vi "GUI_HTT_MultiCamDriveDepletion.vi"() -> ()   [LabVIEW 2020]
uses:
  Shared/GUI_Template/GUI_master/tcp_new_data_event.ctl
  Shared/GUI_Template/GUI_master/tcp new data cluster.ctl
  General GUIs/Device GUIs/GUI_Cameras/Controls/Crosshair type def.ctl
  <userlib>/_OpenG.lib/array/array.llb/Filter 1D Array with Scalar (String)__ogtk.vi
panel:
  out "image1 3":T1(plugin-control)
  out "image1 2":T1(plugin-control)
  out "image1":T1(plugin-control)
  out "String 3":string="x1\ny1\nx2\ny2"
  out "String 2":string="x1\ny1\nx2\ny2"
  out "String":string="x1\ny1\nx2\ny2"
  in  "visibility":bool=TRUE
  out "appended array":string[](array[string]) caption="XH"
  out "appended array 6":string[](array[string]) caption="XH"
  out "appended array 4":string[](array[string]) caption="XH"
  in  "UDP error message":string
  out "tcp data event 2":T2
  out "error IO 2":errorcluster
  in  "Color Box":u32(colorbox)
  in  "TargetSize.Y::4":dbl=45.0 caption="y" min=2.0 max=3000.0 format="%#_6f"
  in  "TargetSize.X::4":dbl=47.0 caption="x" min=2.0 max=3000.0 format="%#_6f"
  in  "TargetSize.Y::3":dbl=163.0 caption="y" min=2.0 max=3000.0 format="%#_6f"
  in  "TargetSize.X::3":dbl=152.0 caption="x" min=2.0 max=3000.0 format="%#_6f"
  in  "TargetSize.Y::2":dbl=74.0 caption="y" min=2.0 max=3000.0 format="%#_6f"
  in  "TargetSize.X::2":dbl=75.0 caption="x" min=2.0 max=3000.0 format="%#_6f"
  in  "active cams":string
  out "CCDs":string[](array[string])
  out "Cameras":T3
  in  "Target.Y::4":dbl=45.0 caption="y" min=0.0 max=2000.0 format="%#_6f"
  in  "Target.X::4":dbl=47.0 caption="x" min=0.0 max=2000.0 format="%#_6f"
  in  "Target.Y::3":dbl=163.0 caption="y" min=0.0 max=2000.0 format="%#_6f"
  in  "Target.X::3":dbl=152.0 caption="x" min=0.0 max=2000.0 format="%#_6f"
  in  "Target.Y::2":dbl=74.0 caption="y" min=0.0 max=2000.0 format="%#_6f"
  in  "Target.X::2":dbl=75.0 caption="x" min=0.0 max=2000.0 format="%#_6f"
  out "error out":errorcluster
  in  "triggerdelay::4":dbl=0.001 caption="triggerdelay" min=0.0 max=1000000.0 format="%_4p"
  in  "triggerdelay::3":dbl=0.001 caption="triggerdelay" min=0.0 max=1000000.0 format="%_4p"
  in  "triggerdelay::2":dbl=0.001 caption="triggerdelay" min=0.0 max=100000.0 format="%_4p"
  in  "centroidy::5":dbl=0.001 caption="centroid y" min=0.0 max=0.0 format="%_4f"
  in  "centroidx::5":dbl=0.001 caption="centroid x" min=0.0 max=0.0 format="%_4f"
  in  "trigger::4":bool caption="Trigger"
  in  "centroidy::4":dbl=0.001 caption="centroid y" min=0.0 max=0.0 format="%_4f"
  in  "centroidx::4":dbl=0.001 caption="centroid x" min=0.0 max=0.0 format="%_4f"
  in  "exposure::4":dbl=0.001 caption="exposure" min=0.0 max=1000000.0 format="%_4p"
  out "image::4":T1(plugin-control) caption="HTT-MagCam-02"
  in  "GUIdevice 4":string="BellaCam24_4_dep4"
  in  "trigger::3":bool caption="Trigger"
  in  "centroidy::3":dbl=0.001 caption="centroid y" min=0.0 max=0.0 format="%_4f"
  in  "centroidx::3":dbl=0.001 caption="centroid x" min=0.0 max=0.0 format="%_4f"
  in  "exposure::3":dbl=0.001 caption="exposure" min=0.0001 max=1.0 format="%_4p"
  out "image::3":T1(plugin-control) caption="HTT-MagCam-03"
  in  "GUIdevice 3":string="BellaCam13_2_dep3"
  in  "trigger::2":bool caption="Trigger"
  in  "centroidy::2":dbl=0.001 caption="centroid y" min=0.0 max=0.0 format="%_4f"
  in  "centroidx::2":dbl=0.001 caption="centroid x" min=0.0 max=0.0 format="%_4f"
  in  "exposure::2":dbl=0.001 caption="exposure" min=1e-05 max=1.0 format="%_4p"
  out "image::2":T1(plugin-control) caption="HTT-MagCam-04"
  in  "GUIdevice 2":string="BellaCam24_2_dep2"
  out "tcp data event":T2
  in  "Refresh Button":bool caption="Update Crosshairs"
  in  "Select device":string(combo)="FrogHPD"
  in  "stop":bool
  in  "GUIdevice 1":string="HPD_CCD"
  # "XHair location"
  # "XHair location"
  # "XHair size"
  # "XHair size"
  # "XHair location"
  # "XHair size"
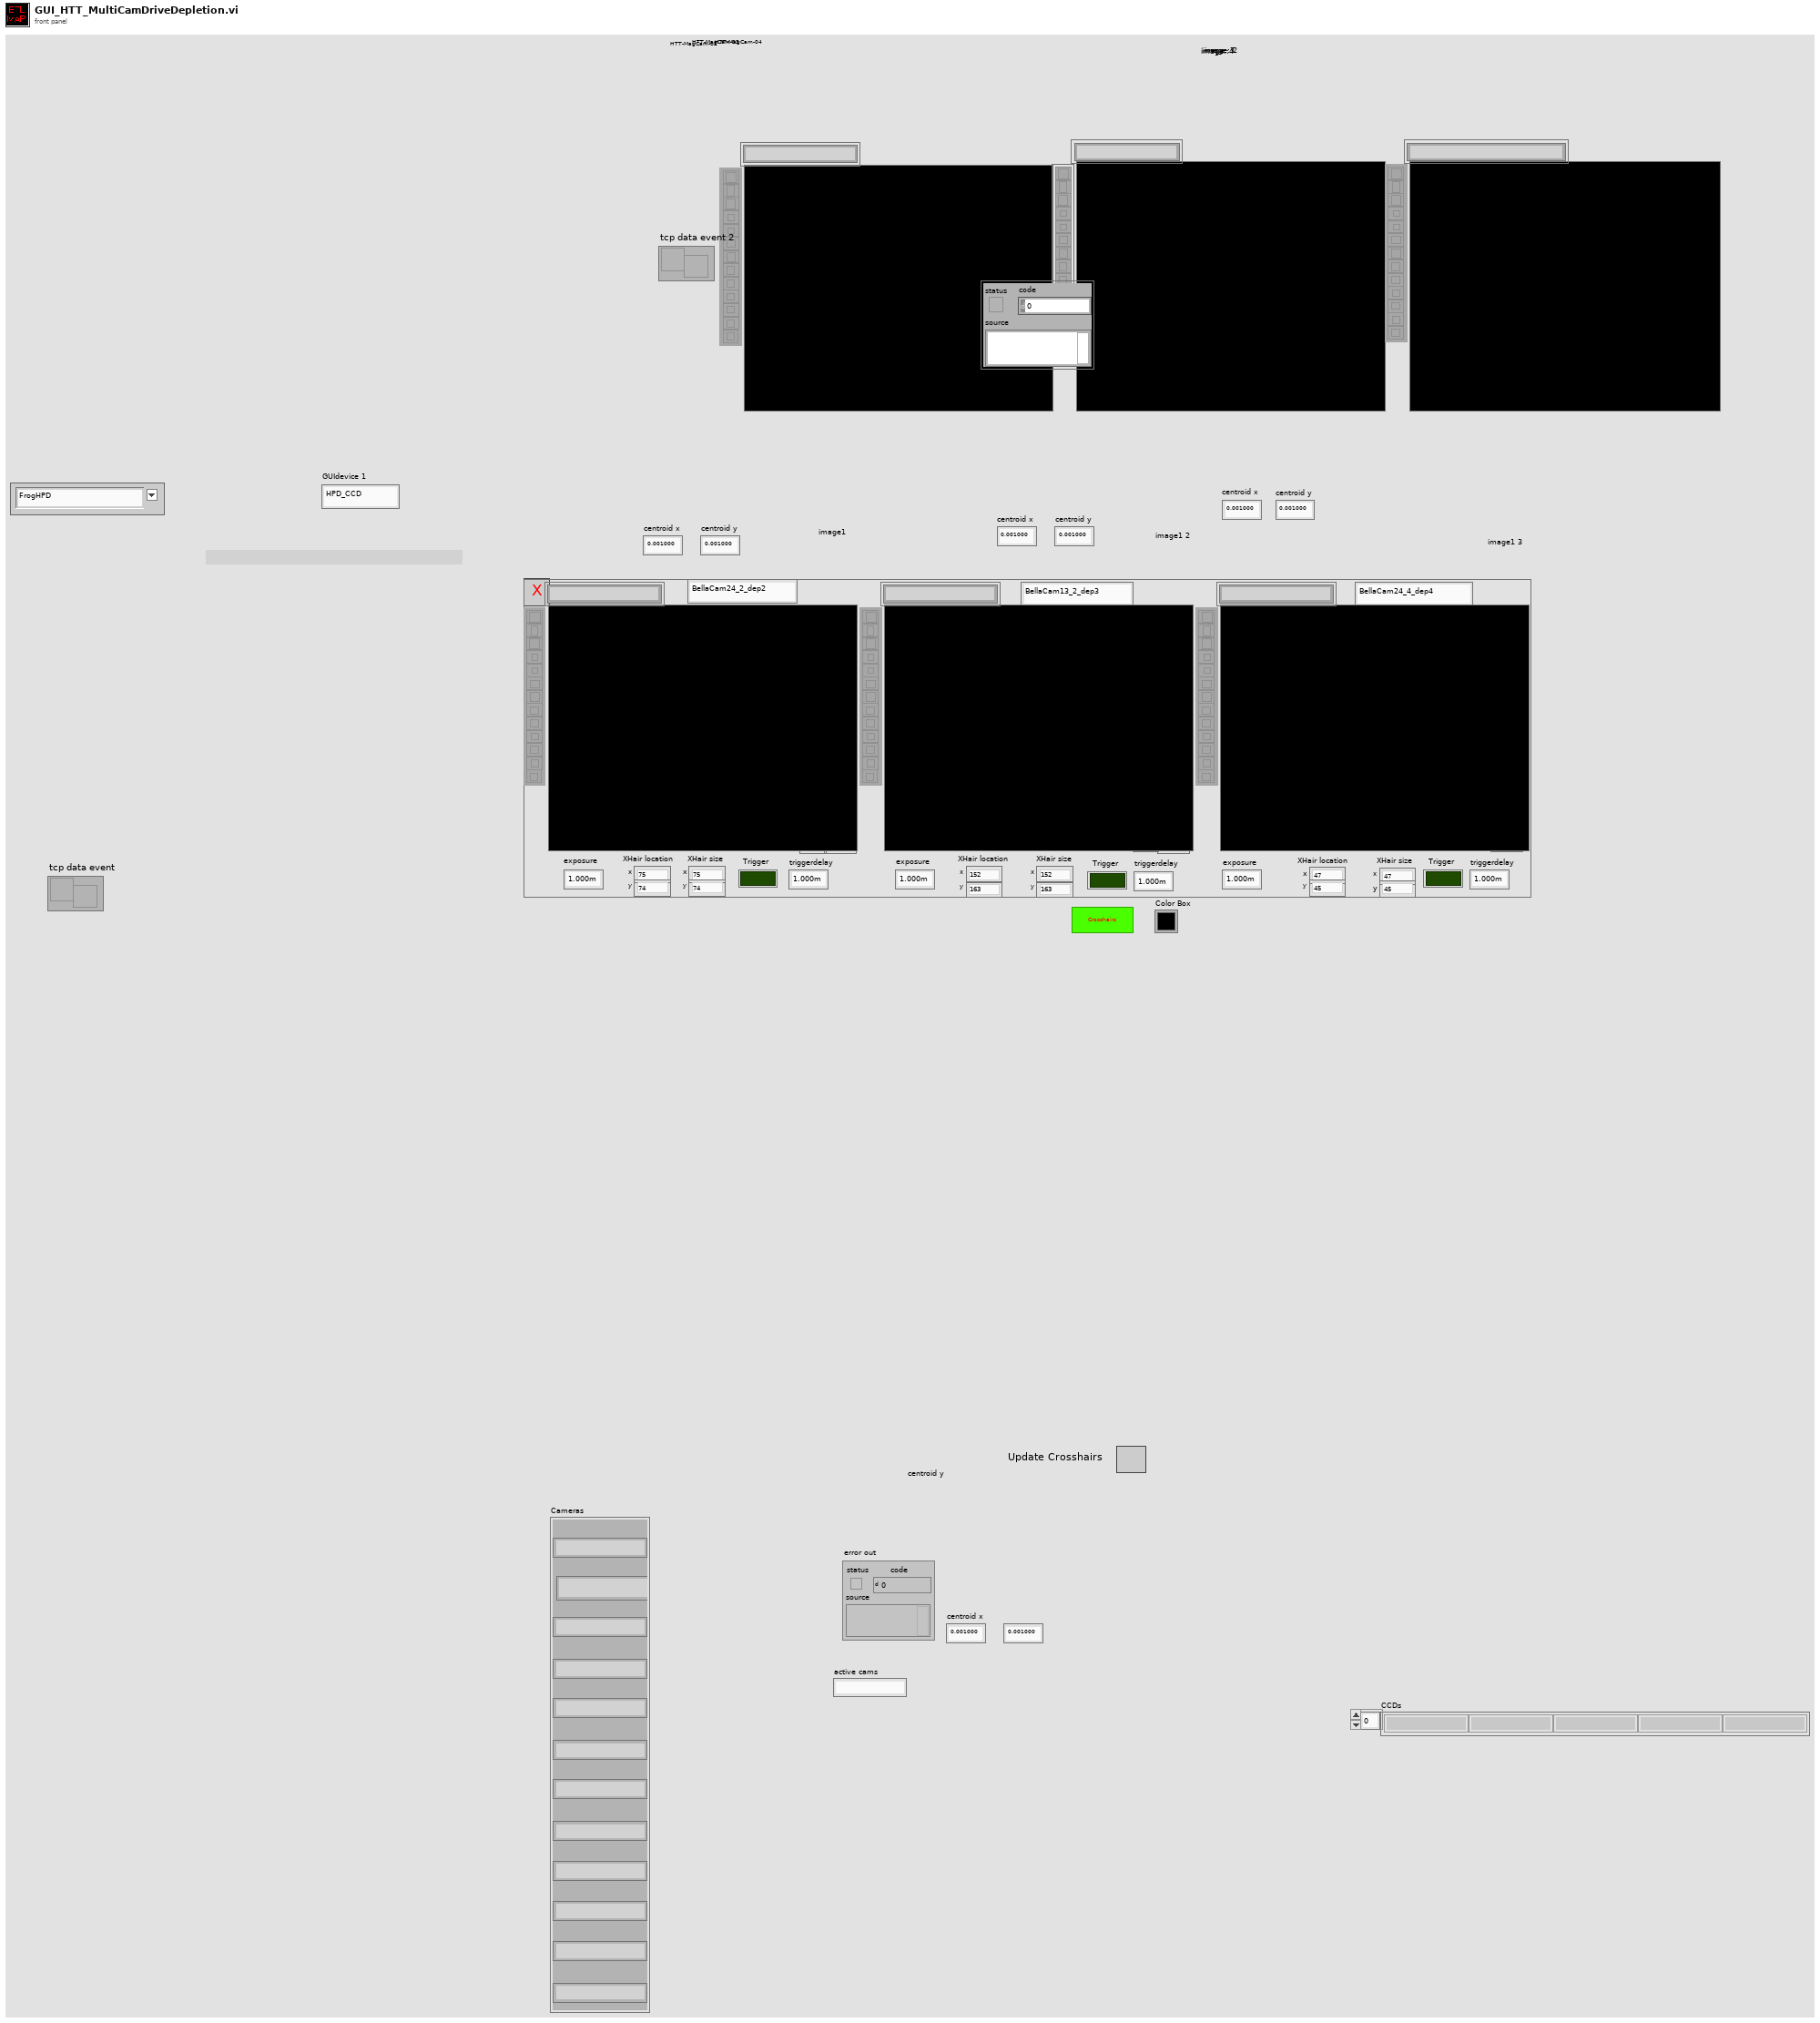
[diagram p1: front panel]
types:
  T1 = typedef "IMAQ Image.ctl" = refnum<image>
  T2 = typedef "tcp_new_data_event.ctl" = refnum<user-event>
  T3 = cluster{"[0]":string, "[1]":string, "[2]":string, "[3]":string, "[4]":string, "[5]":string, "[6]":string, "[7]":string, "[8]":string, "[8] 2":string, "[8] 3":string, "[8] 4":string}
  T4 = typedef "Image Type" = u32
  T5 = cluster{"Target.X::2":refnum<vi>, "Target.Y::2":refnum<vi>}
  T6 = cluster{"Target.X::3":refnum<vi>, "Target.Y::3":refnum<vi>}
  T7 = cluster{"Target.X::4":refnum<vi>, "Target.Y::4":refnum<vi>}
  T8 = cluster{"TargetSize.X::2":refnum<vi>, "TargetSize.Y::2":refnum<vi>}
  T9 = cluster{"TargetSize.X::3":refnum<vi>, "TargetSize.Y::3":refnum<vi>}
  T10 = cluster{"TargetSize.X::4":refnum<vi>, "TargetSize.Y::4":refnum<vi>}
  T11 = cluster{"Target.X::4":refnum<vi>, "Target.Y::4":refnum<vi>}[]
  T12 = cluster{"TargetSize.X::4":refnum<vi>, "TargetSize.Y::4":refnum<vi>}[]
  T13 = cluster{"[0]":string, "[1]":string, "[2]":string, "[3]":string, "[4]":string, "[5]":string, "[6]":string, "[7]":string, "[8]":string, "[9]":string, "[10]":string, "[11]":string}
  T14 = typedef "Crosshair type def.ctl" = cluster{"Draw":bool, "Target":cluster{"x":dbl, "y":dbl}, "Size":cluster{"x":dbl, "y":dbl}, "Angle":dbl, "Color":u32, "Thickness":u8, "CrosshairLabel":string}
  T15 = cluster{"Left":i32, "Top":i32, "Right":i32, "Bottom":i32}
  T16 = enum32{"invalid app kind", "Development System", "Run Time System", "Student Edition", "Embedded LabVIEW", "Evaluation", "Custom"}
  T17 = typedef "tcp new data cluster.ctl" = cluster{"EventEnum":enum16{"new data", "connection status update"}, "Device name":string}
  T18 = enum32{"Invalid", "Standard", "Closed", "Hidden", "Minimized", "Maximized"}
  T19 = cluster{"Core":cluster{"Current VI Reference":refnum<vi>, "Close Panel on Exit?":bool}, "Your Boolean data":bool, "active cams":string, "SuperGUI":cluster{"STOP queue":refnum<queue>, "SuperGUI ref":refnum<vi>}}
  T20 = cluster{"STOP queue":refnum<queue>, "SuperGUI ref":refnum<vi>}
  T21 = cluster{"Current VI Reference":refnum<vi>, "Close Panel on Exit?":bool}
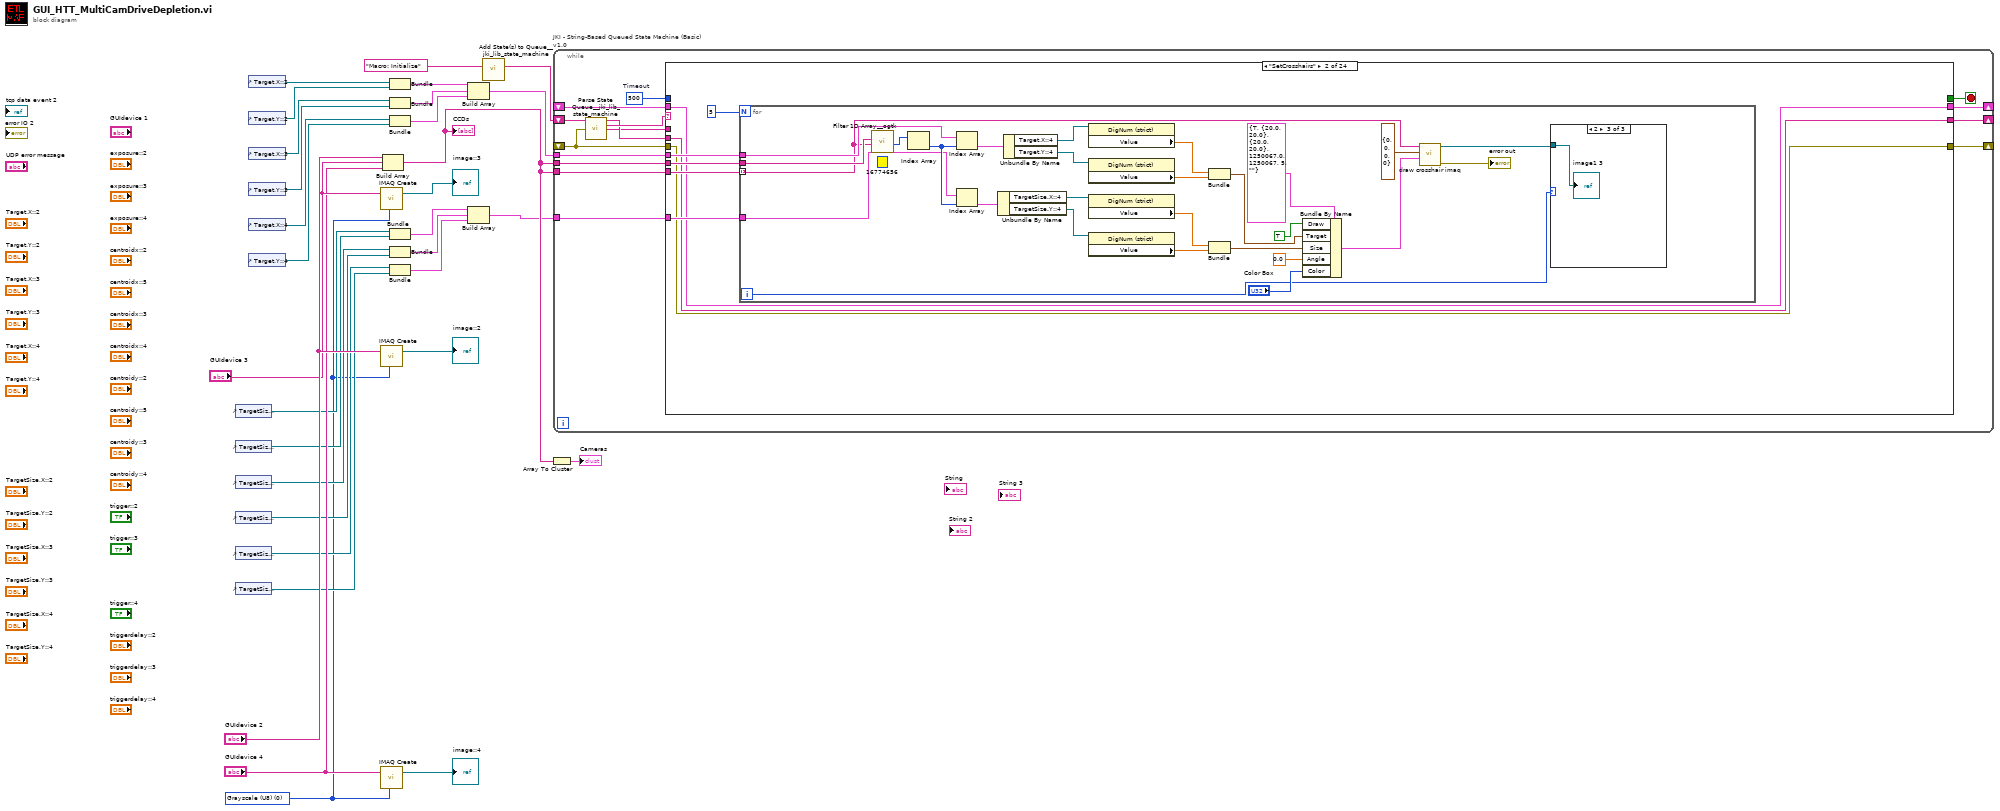
[diagram p0: block diagram]
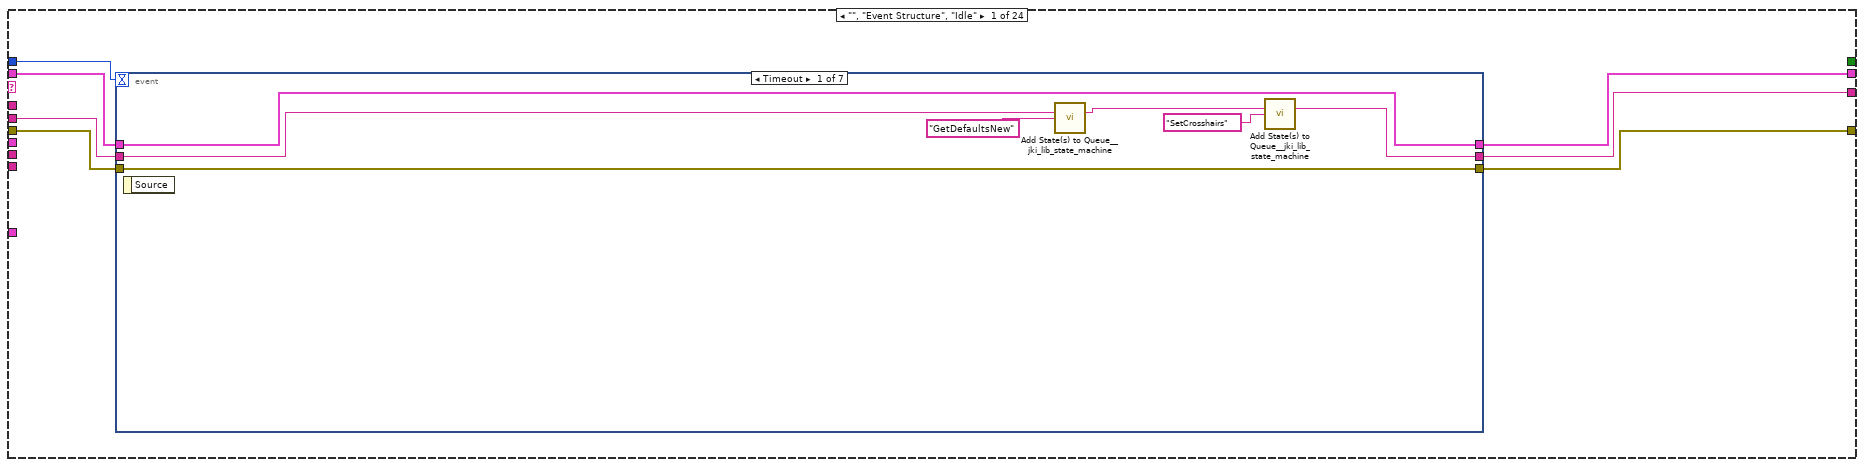
[diagram p2: hidden frame]
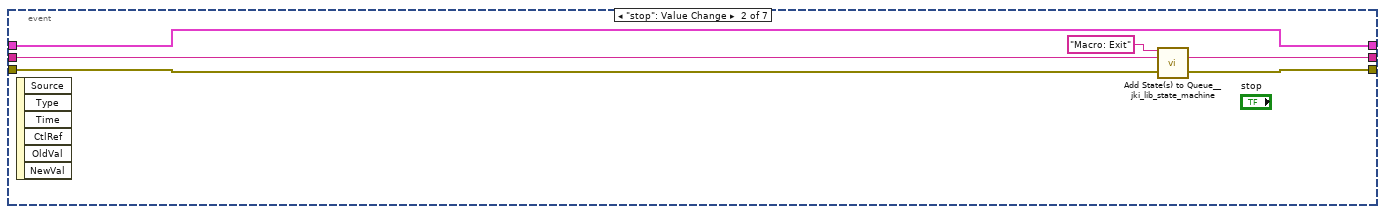
[diagram p3: hidden frame]
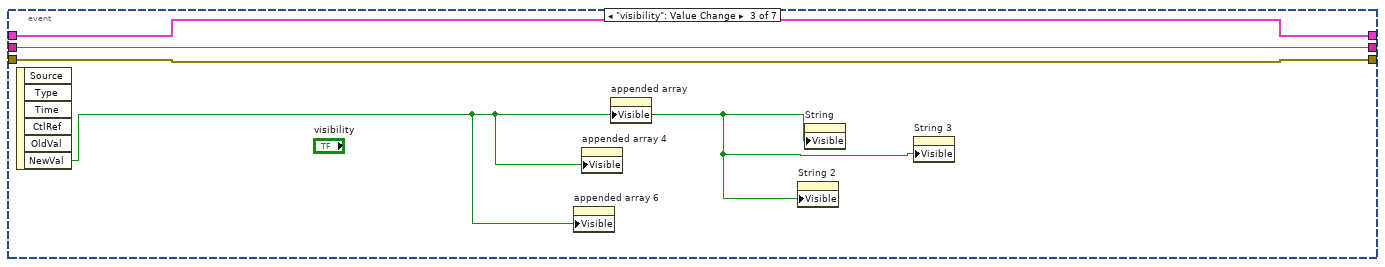
[diagram p4: hidden frame]
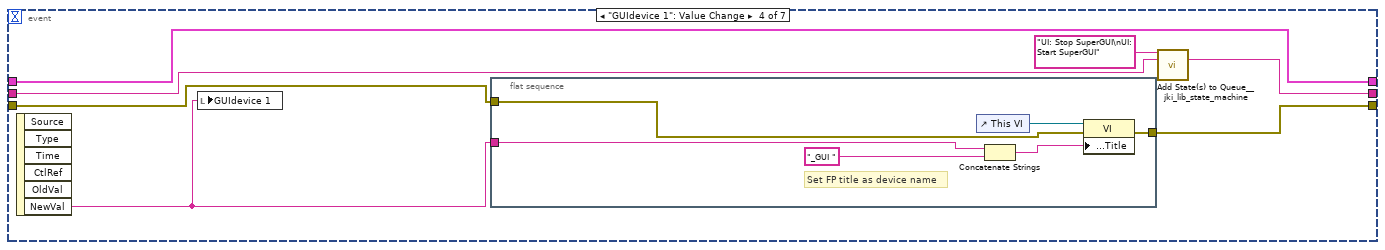
[diagram p5: hidden frame]
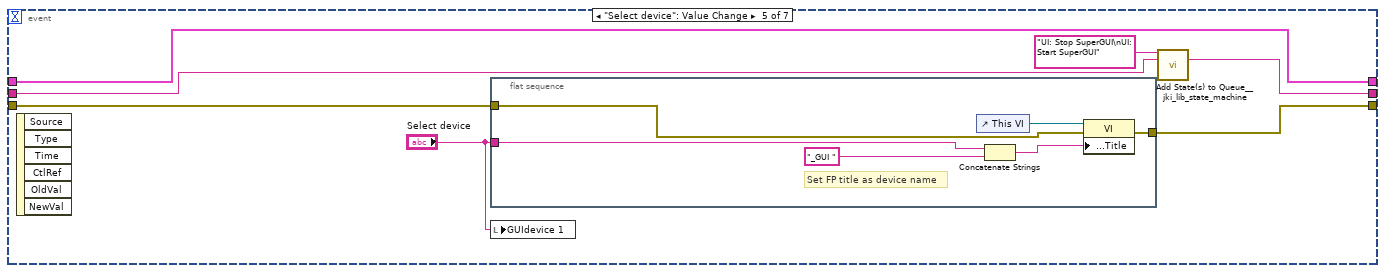
[diagram p6: hidden frame]
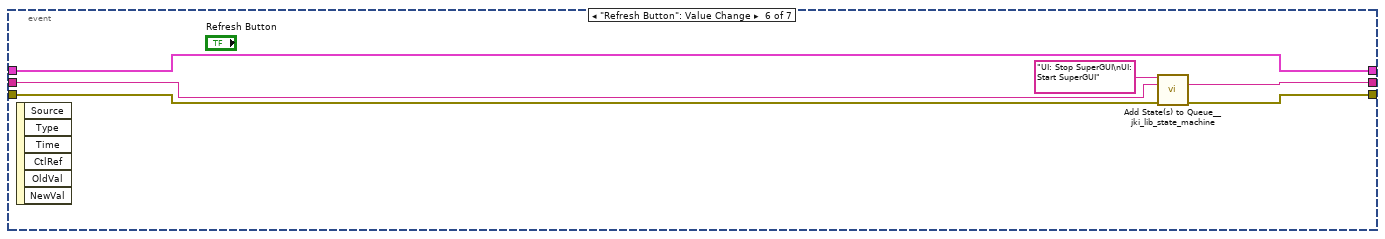
[diagram p7: hidden frame]
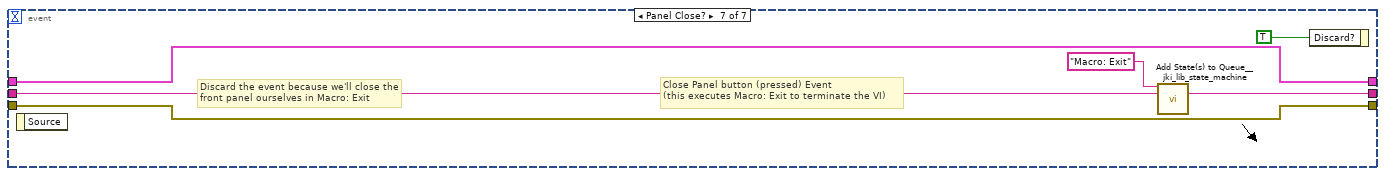
[diagram p8: hidden frame]
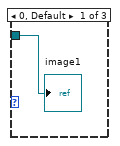
[diagram p9: hidden frame]
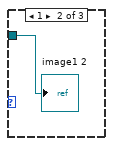
[diagram p10: hidden frame]
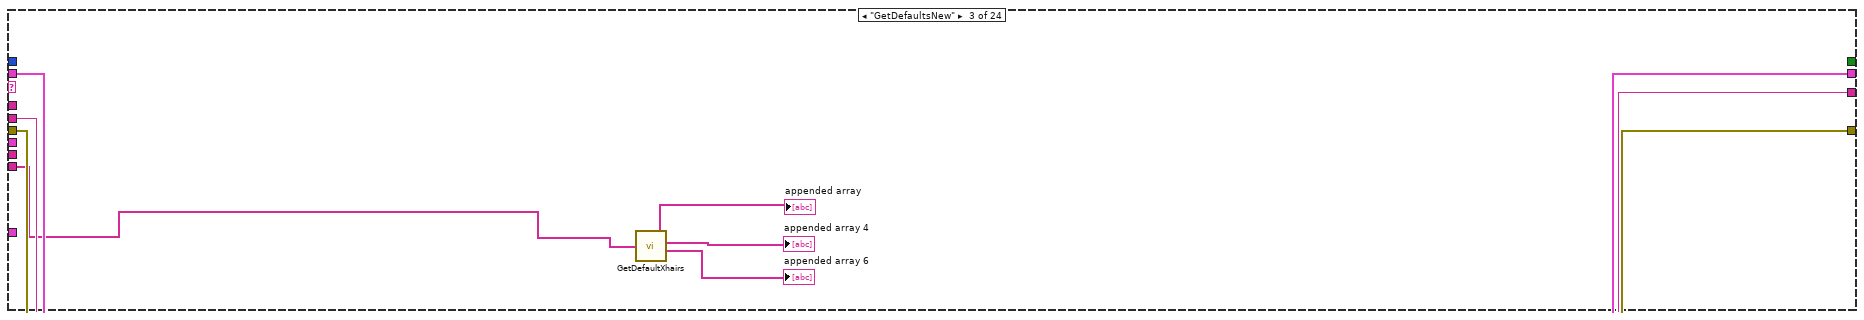
[diagram p11: hidden frame]
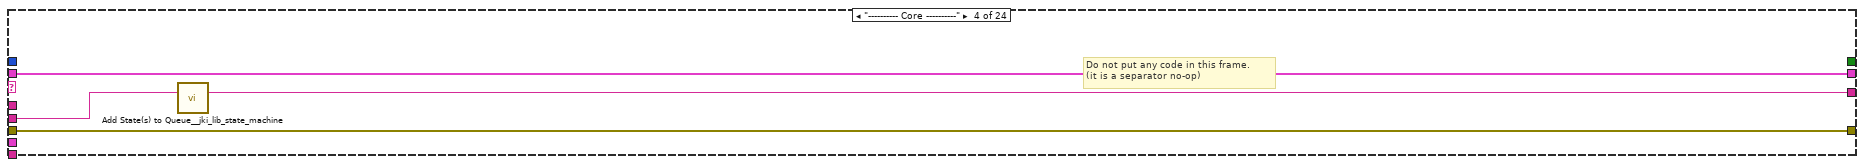
[diagram p12: hidden frame]
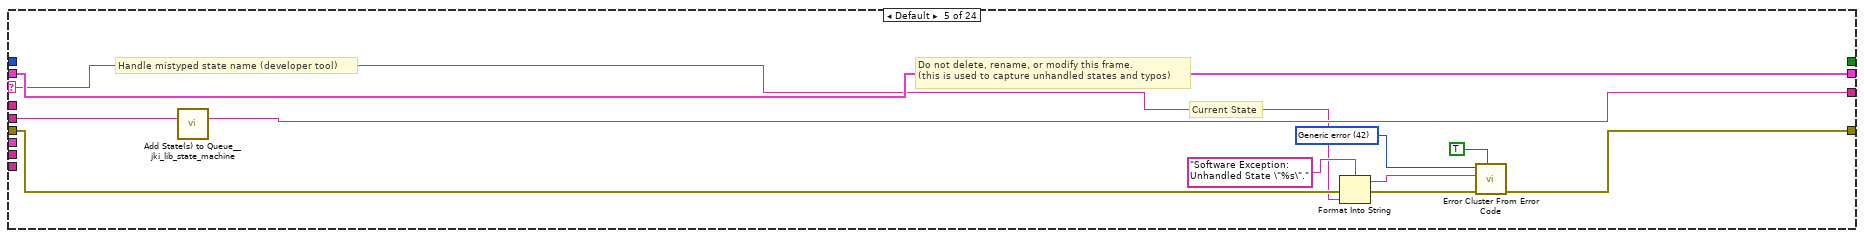
[diagram p13: hidden frame]
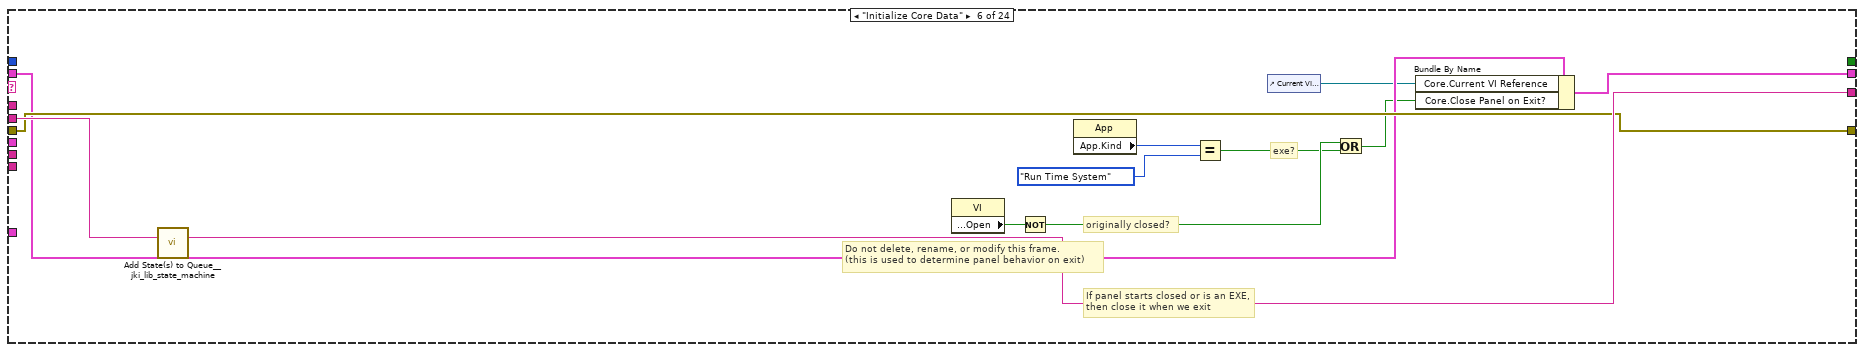
[diagram p14: hidden frame]
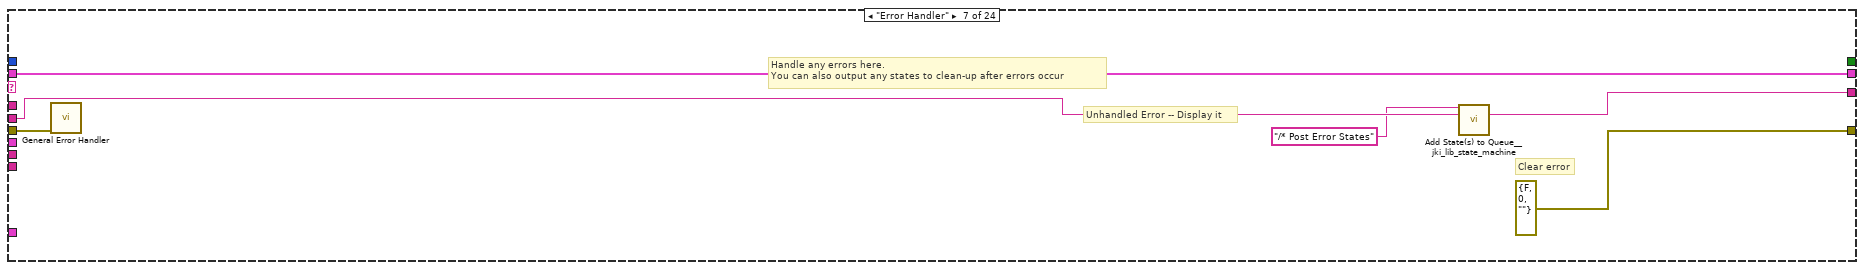
[diagram p15: hidden frame]
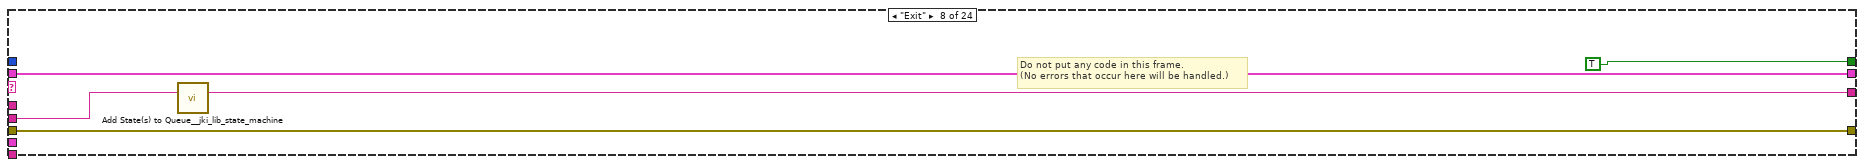
[diagram p16: hidden frame]
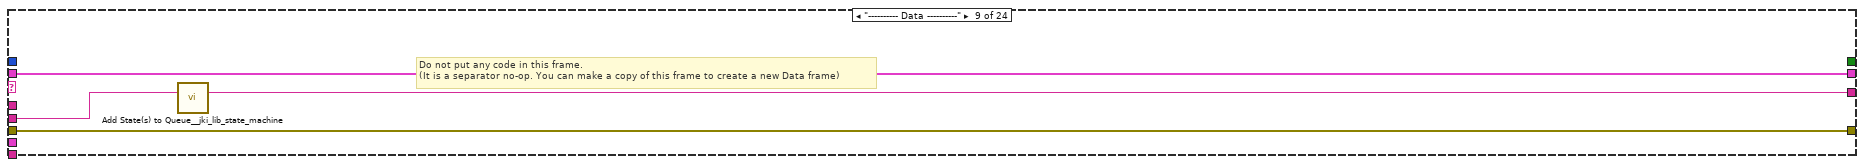
[diagram p17: hidden frame]
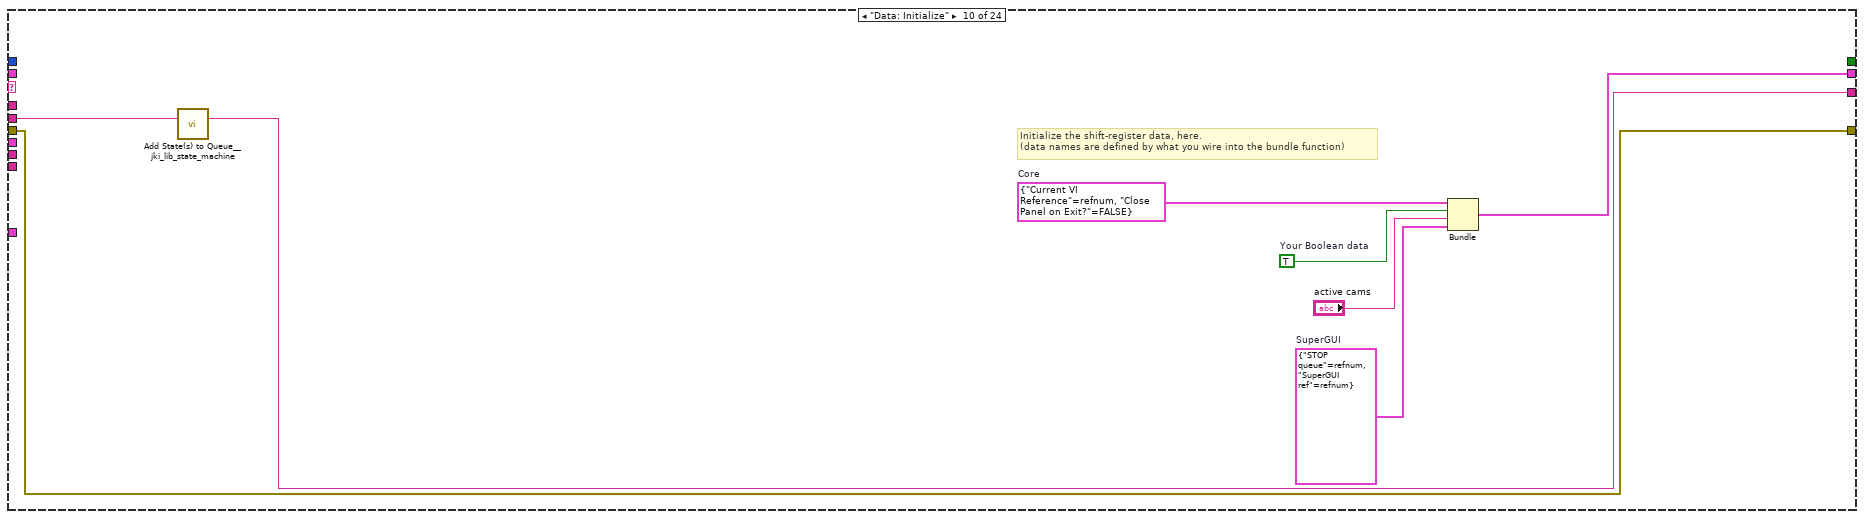
[diagram p18: hidden frame]
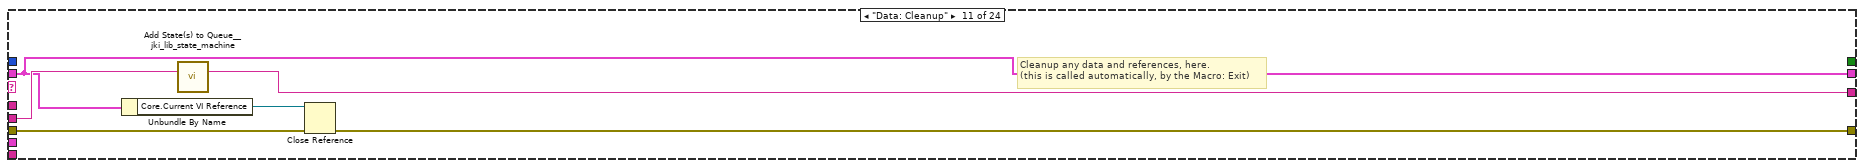
[diagram p19: hidden frame]
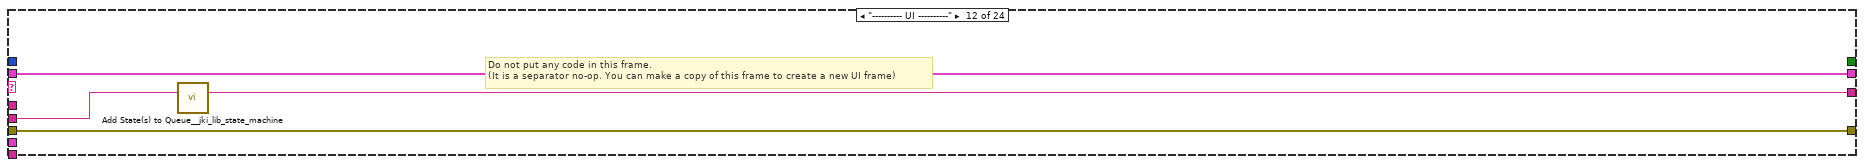
[diagram p20: hidden frame]
diagram:
  w1 = T4 0 items=["Grayscale (U8)", "Grayscale (I16)", "Grayscale (SGL)", "Complex (CSG)", "RGB (U32)", "HSL (U32)", "RGB (U64)", "Grayscale (U16)"] ("Image Type")
  n1 = control-ref of="TargetSize.X::2"() -> (w11:refnum<vi>)
  n2 = control-ref of="TargetSize.Y::2"() -> (w10:refnum<vi>)
  n3 = control-ref of="TargetSize.X::3"() -> (w9:refnum<vi>)
  n4 = control-ref of="TargetSize.Y::3"() -> (w8:refnum<vi>)
  n5 = control-ref of="TargetSize.X::4"() -> (w7:refnum<vi>)
  n6 = control-ref of="TargetSize.Y::4"() -> (w6:refnum<vi>)
  n7 = control-ref of="Target.X::2"() -> (w26:refnum<vi>)
  n8 = control-ref of="Target.Y::2"() -> (w25:refnum<vi>)
  n9 = control-ref of="Target.X::3"() -> (w24:refnum<vi>)
  n10 = control-ref of="Target.Y::3"() -> (w23:refnum<vi>)
  n11 = control-ref of="Target.X::4"() -> (w22:refnum<vi>)
  n12 = control-ref of="Target.Y::4"() -> (w21:refnum<vi>)
  n13 = call "IMAQ Create"("Image Name"="GUIdevice 3", "Image Type"=w1) -> ("New Image"=→"image::3":T1)  [unwired: 3 in, 1 out]
  n14 = call "IMAQ Create"("Image Name"="GUIdevice 2", "Image Type"=w1) -> ("New Image"=→"image::2":T1)  [unwired: 3 in, 1 out]
  n15 = call "IMAQ Create"("Image Name"="GUIdevice 4", "Image Type"=w1) -> ("New Image"=→"image::4":T1)  [unwired: 3 in, 1 out]
  n16 = Build Array("GUIdevice 2", "GUIdevice 3", "GUIdevice 4") -> (w12:string[])
  "CCDs" <- w12
  n17 = Bundle("Target.X::2"=w26, "Target.Y::2"=w25) -> (w20:T5)  [unwired: 1 in]
  n18 = Bundle("Target.X::3"=w24, "Target.Y::3"=w23) -> (w19:T6)  [unwired: 1 in]
  n19 = Bundle("Target.X::4"=w22, "Target.Y::4"=w21) -> (w18:T7)  [unwired: 1 in]
  n20 = Bundle("TargetSize.X::2"=w11, "TargetSize.Y::2"=w10) -> (w5:T8)  [unwired: 1 in]
  n21 = Bundle("TargetSize.X::3"=w9, "TargetSize.Y::3"=w8) -> (w4:T9)  [unwired: 1 in]
  n22 = Bundle("TargetSize.X::4"=w7, "TargetSize.Y::4"=w6) -> (w3:T10)  [unwired: 1 in]
  n23 = Build Array(w20, w19, w18) -> (w17:T11)
  n24 = Build Array(w5, w4, w3) -> (w2:T12)
  n25 = call <vilib>:"Add State(s) to Queue__jki_lib_state_machine.vi"("State(s) in (\"\")"="Macro: Initialize") -> ("States Out"=w31:string)  [unwired: 14 in]
  n26 = Array To Cluster(array=w12) -> (cluster=→"Cameras":T13)
  n27 = while "JKI - String-Based Queued State Machine (Basic) v1.0" {
    shift-right: [w39] -> _
    shift-left: _ -> [w36]
    shift-right: [w42] -> _
    shift-left: _ -> [w37]
    shift-right: [w41] -> _
    shift-left: w31 -> [w43]
    tunnel: w17 -> [w33]
    tunnel: w12 -> [w34]
    tunnel: w12 -> [w35]
    tunnel: w2 -> [w32]
    stop <- w40 stop-if-true
    w38 = 500  # Timeout
    n28 = call <vilib>:"Parse State Queue__jki_lib_state_machine.vi"("State Queue"=w43, "Error In (no error)"=w37) -> ("Remaining States"=w45:string, "Current State"=w46:string, "Arguments"=w44:string)  [unwired: 11 in]
    n29 = case shown="\"SetCrosshairs\"" w46 {
      selector: w46 -> [_ _ _ _ w156 _ _ _ _ _ _ _ _ _ _ _ _ _ _ _ _ _ _ _]
      tunnel: w45 -> [w53 w109 w150 w155 w160 w178 w184 w189 w193 w201 w207 w211 w218 w226 w261 w269 w275 w286 w312 w317 w327 w331 w335 w339]
      tunnel: w44 -> [_ _ _ _ _ _ _ _ _ _ _ _ _ _ _ _ w270 w280 _ _ _ _ _ _]
      tunnel: w36 -> [w51 w110 w151 w152 w158 w169 w181 w187 w190 _ w202 w208 w216 w224 w252 w264 w273 w282 w309 w314 w324 w328 w332 w336]
      tunnel: [w50 w108 w149 w153 w162 w175 errorcluster {"status"=FALSE, "code"=0, "source"=""} ("error out") w186 w191 w198 w203 w209 w214 w221 w245 w262 w271 w283 w310 w315 w325 w329 w333 w337] -> w42
      tunnel: w37 -> [w49 w108 w149 w153 w161 w175 w180 w186 w191 w198 w204 w209 w215 w222 w246 w263 w272 w284 w310 w315 w325 w329 w333 w337]
      tunnel: [w52 w109 w150 w154 w159 w177 w183 w188 w192 w200 w206 w210 w217 w225 w260 w268 w274 w285 w311 w316 w326 w330 w334 w338] -> w41
      tunnel: [_ _ _ _ _ _ _ TRUE _ _ _ _ _ _ _ _ _ _ _ _ _ _ _ _] -> w40
      tunnel: [w48 w110 w151 w152 w158 w176 w181 w187 w190 w199 w202 w208 w216 w224 w251 w264 w273 w282 w309 w314 w324 w328 w332 w336] -> w39
      tunnel: w38 -> [w47 _ _ _ _ _ _ _ _ _ _ _ _ _ _ _ _ _ _ _ _ _ _ _]
      tunnel: w35 -> [_ w112 w148 _ _ _ _ _ _ _ _ _ _ _ _ _ _ _ _ _ _ _ _ _]
      tunnel: w34 -> [_ w113 _ _ _ _ _ _ _ _ _ _ _ _ _ _ _ _ _ _ _ _ _ _]
      tunnel: w33 -> [_ w114 _ _ _ _ _ _ _ _ _ _ _ _ _ _ _ _ _ _ _ _ _ _]
      tunnel: w32 -> [_ w111 _ _ _ _ _ _ _ _ _ _ _ _ _ _ _ _ _ _ _ _ _ _]
      frame "", "Event Structure", "Idle" {
        n30 = event shown="[0] Timeout" {
          selector: _ -> [_ _ _ _ _ _ _]
          dyn-events: _ -> [_ _ _ _ _ _ _]
          timeout: w47 -> [_ _ _ _ _ _ _]
          tunnel: w53 -> [w56 w63 w67 w73 w85 w98 w106]
          tunnel: [w60 w62 w67 w72 w84 w97 w105] -> w52
          tunnel: w51 -> [w58 w65 w69 w76 w89 w100 w103]
          tunnel: [w59 w64 w68 w74 w87 w99 w104] -> w50
          tunnel: w49 -> [w59 w64 w68 w75 w88 w99 w104]
          tunnel: [w58 w65 w69 w76 w89 w100 w103] -> w48
          event Timeout {
            n31 = event-data() -> ()  [unwired: 1 in, 1 out]
            n32 = call <vilib>:"Add State(s) to Queue__jki_lib_state_machine.vi"("State(s) in (\"\")"=w56, "State(s) at Back (\"\")"="GetDefaultsNew") -> ("States Out"=w54:string)  [unwired: 13 in]
            n33 = call <vilib>:"Add State(s) to Queue__jki_lib_state_machine.vi"("State(s) in (\"\")"=w54, "State(s) at Back (\"\")"="SetCrosshairs") -> ("States Out"=w60:string)  [unwired: 13 in]
          }
          event "stop": Value Change {
            n34 = event-data() -> ()  [unwired: 1 in, 6 out]
            n35 = call <vilib>:"Add State(s) to Queue__jki_lib_state_machine.vi"("State(s) in Front (\"\")"="Macro: Exit", "State(s) in (\"\")"=w63) -> ("States Out"=w62:string)  [unwired: 13 in]
          }
          event "visibility": Value Change {
            n36 = event-data() -> ("NewVal"=w66:bool)  [unwired: 1 in, 5 out]
            n37 = property on="appended array 6" class="Arr (strict)"("Visible"=w66) -> ()  [unwired: 2 in, 2 out]
            n38 = property on="appended array 4" class="Arr (strict)"("Visible"=w66) -> ()  [unwired: 2 in, 2 out]
            n39 = property on="appended array" class="Arr (strict)"("Visible"=w66) -> ()  [unwired: 2 in, 2 out]
            n40 = property on="String 2" class="Str"("Visible"=w66) -> ()  [unwired: 2 in, 2 out]
            n41 = property on="String" class="Str"("Visible"=w66) -> ()  [unwired: 2 in, 2 out]
            n42 = property on="String 3" class="Str"("Visible"=w66) -> ()  [unwired: 2 in, 2 out]
          }
          event "GUIdevice 1": Value Change {
            n43 = event-data() -> ("NewVal"=w70:string)  [unwired: 1 in, 5 out]
            n44 = local write "GUIdevice 1"(w70) -> ()
            n45 = flat-sequence {
              tunnel: [w79] -> w74
              tunnel: w75 -> [w78]
              tunnel: w70 -> [w77]
              frame #0 {
                # "Set FP title as device name"
                n46 = control-ref of="This VI"() -> (w82:refnum<vi>)
                n47 = Concatenate Strings(w77, "_GUI ") -> (w81:string)
                n48 = property class="VI"(reference=w82, error in=w78, "Front Panel.Title"=w81) -> (error out=w79:errorcluster)  [unwired: 1 out]
              }
            }
            n49 = call <vilib>:"Add State(s) to Queue__jki_lib_state_machine.vi"("State(s) in Front (\"\")"="UI: Stop SuperGUI\nUI: Start SuperGUI", "State(s) in (\"\")"=w73) -> ("States Out"=w72:string)  [unwired: 13 in]
          }
          event "Select device": Value Change {
            n50 = event-data() -> ()  [unwired: 1 in, 6 out]
            n51 = flat-sequence {
              tunnel: [w92] -> w87
              tunnel: w88 -> [w91]
              tunnel: "Select device" -> [w90]
              frame #0 {
                # "Set FP title as device name"
                n52 = control-ref of="This VI"() -> (w95:refnum<vi>)
                n53 = Concatenate Strings(w90, "_GUI ") -> (w94:string)
                n54 = property class="VI"(reference=w95, error in=w91, "Front Panel.Title"=w94) -> (error out=w92:errorcluster)  [unwired: 1 out]
              }
            }
            n55 = local write "GUIdevice 1"("Select device") -> ()
            n56 = call <vilib>:"Add State(s) to Queue__jki_lib_state_machine.vi"("State(s) in Front (\"\")"="UI: Stop SuperGUI\nUI: Start SuperGUI", "State(s) in (\"\")"=w85) -> ("States Out"=w84:string)  [unwired: 13 in]
          }
          event "Refresh Button": Value Change {
            n57 = event-data() -> ()  [unwired: 1 in, 6 out]
            n58 = call <vilib>:"Add State(s) to Queue__jki_lib_state_machine.vi"("State(s) in Front (\"\")"="UI: Stop SuperGUI\nUI: Start SuperGUI", "State(s) in (\"\")"=w98) -> ("States Out"=w97:string)  [unwired: 13 in]
          }
          event Panel Close? {
            # "Discard the event because we'll close the front panel ourselves in Macro: Exit"
            # "Close Panel button (pressed) Event\n(this executes Macro: Exit to terminate the VI)"
            n59 = event-data() -> ()  [unwired: 1 in, 1 out]
            n60 = call <vilib>:"Add State(s) to Queue__jki_lib_state_machine.vi"("State(s) in Front (\"\")"="Macro: Exit", "State(s) in (\"\")"=w106) -> ("States Out"=w105:string)  [unwired: 13 in]
            n61 = event-data("Discard?"=TRUE) -> ()  [unwired: 1 in, 1 out]
          }
        }
      }
      frame "SetCrosshairs" {
        n62 = for {
          N: 5 -> [_]
          tunnel: w113 -> [w120]
          tunnel: w114 -> [w119]
          tunnel: w111 -> [w118]
          tunnel: w112 -> [w117] mode=indexing
          i -> [w116]
          (unwired) u32 16774656 ("Color")
          n63 = call-poly <userlib>:"Filter 1D Array__ogtk.vi"("items to filter"=w117, "array"=w120) -> ("filtered item indices"=w124:i32[])  [unwired: 4 in, 1 out]
          n64 = Index Array(array=w124) -> (element=w127:i32)  [unwired: 1 in]
          n65 = Index Array(array=w119, index=w127) -> (element=w125:T7)
          n66 = Index Array(array=w118, index=w127) -> (element=w128:T10)
          n67 = Unbundle By Name(w128) -> ("TargetSize.X::4"=w129:refnum<vi>, "TargetSize.Y::4"=w130:refnum<vi>)
          n68 = Unbundle By Name(w125) -> ("Target.X::4"=w122:refnum<vi>, "Target.Y::4"=w123:refnum<vi>)
          n69 = property class="DigNum (strict)"(reference=w122) -> ("Value"=w136:dbl)  [unwired: 1 in, 2 out]
          n70 = property class="DigNum (strict)"(reference=w123) -> ("Value"=w137:dbl)  [unwired: 1 in, 2 out]
          n71 = property class="DigNum (strict)"(reference=w129) -> ("Value"=w131:dbl)  [unwired: 1 in, 2 out]
          n72 = property class="DigNum (strict)"(reference=w130) -> ("Value"=w132:dbl)  [unwired: 1 in, 2 out]
          n73 = Bundle("Value"=w136, "Value"=w137) -> (w138:cluster{"Value":dbl, "Value":dbl})  [unwired: 1 in]
          n74 = Bundle("Value"=w131, "Value"=w132) -> (w139:cluster{"Value":dbl, "Value":dbl})  [unwired: 1 in]
          n75 = Bundle By Name(cluster=T14 {"Draw"=TRUE, "Target"={"x"=20.0, "y"=20.0}, "Size"={"x"=20.0, "y"=20.0}, "Angle"=1250067.0, "Color"=1250067, "Thickness"=5, "CrosshairLabel"=""} ("Crosshair"), "Draw"=TRUE, "Target"=w138, "Size"=w139, "Angle"=0.0, "Color"="Color Box") -> (w134:T14)
          n76 = call "draw crosshair imaq.vi"("Crosshair"=w134, "Bounding Rectangle"=T15 {"Left"=0, "Top"=0, "Right"=0, "Bottom"=0}, "image in"=w117) -> ("error out"=→"error out":errorcluster, "image out"=w115:T1)  [unwired: 7 in]
          n77 = case shown="2" w116 {
            tunnel: w115 -> [w142 w143 w144]
            frame 0, Default {
              "image1" <- w142
            }
            frame 1 {
              "image1 2" <- w143
            }
            frame 2 {
              "image1 3" <- w144
            }
          }
        }
      }
      frame "GetDefaultsNew" {
        n78 = call "GetDefaultXhairs.vi"("appended array 2"=w148) -> ("appended array"=→"appended array":string[], "appended array 4"=→"appended array 4":string[], "appended array 6"=→"appended array 6":string[])  [unwired: 1 out]
      }
      frame "---------- Core ----------" {
        # "Do not put any code in this frame.\n(it is a separator no-op)"
        n79 = call <vilib>:"Add State(s) to Queue__jki_lib_state_machine.vi"("State(s) in (\"\")"=w155) -> ("States Out"=w154:string)  [unwired: 14 in]
      }
      frame Default {
        w165 = 42 items=["No error", "Argument error", "Memory is full", "Out of zone", "End of file", "File already open", "Generic file I/O error", "File not found", "File permission error", "Disk is full", "Duplicate path", "Too many files open", "System feature not enabled", "Resource file not found", "Cannot add resource", "Resource not found", "Image not found", "Image memory error", "Pen does not exist", "Config type invalid", "Config token not found", "Config parse error", "Config memory error", "Bad external code format", "Bad external code offset", "External code not present", "Null window", "Destroy window error", "Null menu", "Print aborted", "Bad print record", "Print driver error", "Windows error during printing", "Memory error during printing", "Print dialog error", "Generic print error", "Invalid device refnum", "Device not found", "Device parameter error", "Device unit error", "Cannot open device", "Device call aborted", "Generic error", "Cancelled by user", "Object ID too low", "Object ID too high", "Object not in heap", "Unknown heap", "Unknown object (invalid DefProc)", "Unknown object (DefProc not in table)", "Message out of range", "Invalid (null) method", "Unknown message", "Manager call not supported", "Bad address", "Network operation in progress", "Network operation timed out", "Connection is busy", "Network attribute not supported", "Network error", "Address in use", "System out of memory", "Connection aborted", "Connection refused", "Not connected", "Already connected", "Connection closed", "Initialization error (interapplication manager)", "Bad occurrence", "Wait on unbound occurrence handler", "Occurrence queue overflow", "Datalog type conflict", "Unused", "Unrecognized type (interapplication manager)", "Memory corrupt", "Failed to make temporary DLL", "Old CIN version", "Drag socket not found", "Failed to load drop-object", "Failed to register OLE object", "Failed to release OLE object", "Format specifier type mismatch", "Unknown format specifier", "Too few format specifiers", "Too many format specifiers", "Scan failed", "Newer CIN version", "Error converting to variant", "Runtime menu error", "Password tampered", "Variant attribute not found", "Incompatible variant data type", "Event data is not available", "Event Store is not present", "Occurrence is not found", "Event Queue is not created", "Event info is not available", "Refnum passed is NULL", "Error retrieving Class GUID", "Error retrieving CoClass GUID", "Error retrieving TypeLib GUID.", "Bad built application magic bytes.", "Specific driver is different from the specific driver associated with the Logical Name.", "There is no session opened to the class driver.", "Max Error", "MAX - Error with config objects", "MAX - Error loading configuration", "MAX - Group not supported"]
        # "Current State"
        # "Do not delete, rename, or modify this frame.\n(this is used to capture unhandled states and typos)"
        # "Handle mistyped state name (developer tool)"
        n80 = call <vilib>:"Add State(s) to Queue__jki_lib_state_machine.vi"("State(s) in (\"\")"=w160) -> ("States Out"=w159:string)  [unwired: 14 in]
        n81 = Format Into String(format string="Software Exception: Unhandled State \"%s\"." ("message"), error in=w161, w156) -> (resulting string=w164:string, error out=w163:errorcluster)  [unwired: 1 in]
        n82 = call <vilib>:"Error Cluster From Error Code.vi"("show call chain? (False)"=TRUE, "error in (no error)"=w163, "error message (\"\")"=w164, "error code (0)"=w165) -> ("error out"=w162:errorcluster)  [unwired: 5 in]
      }
      frame "Initialize Core Data" {
        # "Do not delete, rename, or modify this frame.\n(this is used to determine panel behavior on exit)"
        # "originally closed?"
        # "exe?"
        # "If panel starts closed or is an EXE, then close it when we exit"
        n83 = call <vilib>:"Add State(s) to Queue__jki_lib_state_machine.vi"("State(s) in (\"\")"=w178) -> ("States Out"=w177:string)  [unwired: 14 in]
        n84 = property class="VI"() -> ("Front Panel.Open"=w174:bool)  [unwired: 2 in, 2 out]
        n85 = Not(x=w174) -> (.not. x?=w171:bool)
        n86 = property class="App"() -> ("App.Kind"=w173:T16)  [unwired: 2 in, 2 out]
        n87 = Equal?(x=w173, y=T16."Run Time System" ("Application:Kind")) -> (x = y?=w170:bool)
        n88 = control-ref of="Current VI Reference"() -> (w167:refnum<vi>)
        n89 = Or(x=w171, y=w170) -> (x .or. y?=w168:bool)
        n90 = Bundle By Name(cluster=w169, "Core.Current VI Reference"=w167, "Core.Close Panel on Exit?"=w168) -> (w176:T19)
      }
      frame "Error Handler" {
        # "Unhandled Error -- Display it"
        # "Handle any errors here.\nYou can also output any states to clean-up after errors occur"
        # "Clear error"
        n91 = call <vilib>:"General Error Handler.vi"("error in (no error)"=w180) -> ()  [unwired: 10 in, 5 out]
        n92 = call <vilib>:"Add State(s) to Queue__jki_lib_state_machine.vi"("State(s) in Front (\"\")"="/* Post Error States", "State(s) in (\"\")"=w184) -> ("States Out"=w183:string)  [unwired: 13 in]
      }
      frame "Exit" {
        # "Do not put any code in this frame.\n(No errors that occur here will be handled.)"
        n93 = call <vilib>:"Add State(s) to Queue__jki_lib_state_machine.vi"("State(s) in (\"\")"=w189) -> ("States Out"=w188:string)  [unwired: 14 in]
      }
      frame "---------- Data ----------" {
        # "Do not put any code in this frame.\n(It is a separator no-op. You can make a copy of this frame to create a new Data frame)"
        n94 = call <vilib>:"Add State(s) to Queue__jki_lib_state_machine.vi"("State(s) in (\"\")"=w193) -> ("States Out"=w192:string)  [unwired: 14 in]
      }
      frame "Data: Initialize" {
        w194 = T20 {"STOP queue"=refnum, "SuperGUI ref"=refnum}  # SuperGUI
        w195 = T21 {"Current VI Reference"=refnum, "Close Panel on Exit?"=FALSE}  # Core
        w197 = TRUE  # Your Boolean data
        # "Initialize the shift-register data, here.\n(data names are defined by what you wire into the bundle function)"
        n95 = call <vilib>:"Add State(s) to Queue__jki_lib_state_machine.vi"("State(s) in (\"\")"=w201) -> ("States Out"=w200:string)  [unwired: 14 in]
        n96 = Bundle("Core"=w195, "Your Boolean data"=w197, "active cams"="active cams", "SuperGUI"=w194) -> (w199:T19)  [unwired: 1 in]
      }
      frame "Data: Cleanup" {
        # "Cleanup any data and references, here.\n(this is called automatically, by the Macro: Exit)"
        n97 = Unbundle By Name(w202) -> ("Core.Current VI Reference"=w205:refnum<vi>)
        n98 = call <vilib>:"Add State(s) to Queue__jki_lib_state_machine.vi"("State(s) in (\"\")"=w207) -> ("States Out"=w206:string)  [unwired: 14 in]
        n99 = Close Reference(reference=w205, error in (no error)=w204) -> (error out=w203:errorcluster)
      }
      frame "---------- UI ----------" {
        # "Do not put any code in this frame.\n(It is a separator no-op. You can make a copy of this frame to create a new UI frame)"
        n100 = call <vilib>:"Add State(s) to Queue__jki_lib_state_machine.vi"("State(s) in (\"\")"=w211) -> ("States Out"=w210:string)  [unwired: 14 in]
      }
      frame "UI: Initialize" {
        # "Initialize the User Interface, here.\n(this is called automatically, by the Macro: Init)"
        n101 = call <vilib>:"Add State(s) to Queue__jki_lib_state_machine.vi"("State(s) in (\"\")"=w218) -> ("States Out"=w217:string)  [unwired: 14 in]
        n102 = call <userlib>:"Fit VI window to Largest Dec__ogtk.vi"("error in (no error)"=w215) -> ("error out"=w214:errorcluster)  [unwired: 5 in, 1 out]
        n103 = for {
          tunnel: string[] ["Point Grey Camera", "Manta Camera", "Photometrics Cam", "Basler Camera"] -> [w220] mode=indexing
          tunnel: [w219] -> w212 mode=concatenating
          n104 = call "getDevices.vi"("Device Class"=w220) -> ("All Devices"=w219:string[])
        }
        n105 = property on="Select device" class="CmbBox"("Strings[]"=w212) -> ()  [unwired: 2 in, 2 out]
      }
      frame "UI: Get Device Name" {
        # "Initialize the User Interface, here.\n(this is called automatically, by the Macro: Init)"
        n106 = call <vilib>:"Add State(s) to Queue__jki_lib_state_machine.vi"("State(s) in (\"\")"=w226) -> ("States Out"=w225:string)  [unwired: 14 in]
        n107 = First Call?() -> (First Call?: T/F=w223:bool)
        n108 = case shown="True" w223 {
          tunnel: w222 -> [w227 w229]
          tunnel: [w227 w228] -> w221
          frame False {
          }
          frame True {
            n109 = disable-structure "Get Device name from control for vi mode\nand command line arg for exe" shown="RUN_TIME_ENGINE==True" {
              disable-tunnel: w229 -> [w230 w232]
              disable-tunnel: [w230 w231] -> w228
              frame condition #0 (active) {
              }
              frame condition #1 {
                n110 = control-ref of="This Application"() -> (w240:refnum<vi>)
                n111 = property class="App"(reference=w240) -> ("App.Args"=w239:string[])  [unwired: 1 in, 2 out]
                n112 = Index Array(array=w239, index #1=1 ("index")) -> (element #1=w233:string)  [unwired: 2 in, 2 out]
                n113 = Empty String/Path?(string/path=w233) -> (empty?=w237:bool)
                n114 = Concatenate Strings(w233, "_GUI ") -> (w235:string)
                n115 = case shown="False" w237 {
                  tunnel: w233 -> [w241 _]
                  frame False {
                    n116 = local write "GUIdevice 1"(w241) -> ()
                  }
                  frame True {
                  }
                }
                n117 = control-ref of="This VI"() -> (w236:refnum<vi>)
                n118 = property class="VI"(reference=w236, error in=w232, "Front Panel.Title"=w235) -> (error out=w231:errorcluster)  [unwired: 1 out]
              }
            }
          }
        }
      }
      frame "UI: Start SuperGUI" {
        # "create stop queue for supergui and its clones"
        # "x100 abort will be dependent on caller VI\nx80 abort will be independent of caller vi, this will abort vi when labview is closed."
        # "Start SuperGUI asynchronous way"
        n119 = vi-ref "GUI_Master_subvi_reentrant_queues.vi"() -> (w244:refnum<vi>)
        n120 = property class="VI"(reference=w244) -> ("Path"=w243:path)  [unwired: 1 in, 2 out]
        n121 = control-ref of="This Application"() -> (w250:refnum<vi>)
        n122 = Open VI Reference(type specifier VI Refnum (for type only)=refnum<vi> refnum, vi path=w243, options=256) -> (vi reference=w259:refnum<vi>, error out=w258:errorcluster)  [unwired: 3 in]
        n123 = Create User Event(user event datatype=T17 {"EventEnum"=enum."new data", "Device name"="Device name"} ("New Event"), error in=w246) -> (user event=w247:refnum<user-event>, error out=w253:errorcluster)
        "tcp data event" <- w247
        n124 = control-ref of="This VI"() -> (w249:refnum<vi>)
        n125 = register-events(w247) -> ()  [unwired: 2 in, 2 out]
        n126 = call "supergui create stop queue.vi"() -> ("STOP Queue out"=w255:refnum<queue>)  [unwired: 11 in]
        n127 = Current VI's Menubar() -> (w248:refnum<k9>)
        n128 = call-by-ref "Start Asynchronous Call"(reference=w259, error in=w258, "STOP Queue in"=w255, "This Application"=w250, 8:"error in (no error)"=w253, "tcp data event"=w247, "Caller menu reference"=w248, "Caller VI ref"=w249) -> (reference out=w242:refnum<vi>, error out=w245:errorcluster)  [unwired: 5 in, 1 out]
        n129 = Bundle By Name(cluster=w252, "SuperGUI.SuperGUI ref"=w242, "SuperGUI.STOP queue"=w255) -> (w251:T19)
        n130 = call <vilib>:"Add State(s) to Queue__jki_lib_state_machine.vi"("State(s) in (\"\")"=w261) -> ("States Out"=w260:string)  [unwired: 14 in]
      }
      frame "UI: Stop SuperGUI" {
        # "Stop Supergui Clone and wait until it exit properly"
        n131 = call <vilib>:"Add State(s) to Queue__jki_lib_state_machine.vi"("State(s) in (\"\")"=w269) -> ("States Out"=w268:string)  [unwired: 14 in]
        n132 = Unbundle By Name(w264) -> ("SuperGUI.SuperGUI ref"=w266:refnum<vi>, "SuperGUI.STOP queue"=w265:refnum<queue>)
        n133 = Release Queue(queue=w265, error in (no error)=w263) -> (error out=w267:errorcluster)  [unwired: 1 in, 2 out]
        n134 = call-by-ref "Wait On Asynchronous Call"(reference=w266, error in=w267) -> ("error out"=w262:errorcluster)  [unwired: 11 in, 2 out]
      }
      frame "UI: Cursor Set" {
        # "Argument"
        # "Set and Unset Cursor Busy.\n(Usage: \"UI: Cursor Set >> Busy|Idle\")"
        n135 = call <vilib>:"Add State(s) to Queue__jki_lib_state_machine.vi"("State(s) in (\"\")"=w275) -> ("States Out"=w274:string)  [unwired: 14 in]
        n136 = case shown="\"Idle\", Default" w270 {
          tunnel: w272 -> [w277 w279]
          tunnel: [w276 w278] -> w271
          frame "Idle", Default {
            n137 = call <vilib>:"Unset Busy.vi"("error in (no error)"=w277) -> ("error out"=w276:errorcluster)  [unwired: 10 in]
          }
          frame "Busy" {
            n138 = call <vilib>:"Set Busy.vi"("error in (no error)"=w279) -> ("error out"=w278:errorcluster)  [unwired: 9 in, 1 out]
          }
        }
      }
      frame "UI: Front Panel State" {
        # "Argument"
        # "Set Front Panel Open or Closed\n(Usage: \"UI: Front Panel State >> Open|Close\")"
        n139 = call <vilib>:"Add State(s) to Queue__jki_lib_state_machine.vi"("State(s) in (\"\")"=w286) -> ("States Out"=w285:string)  [unwired: 14 in]
        n140 = Unbundle By Name(w282) -> ("Core.Current VI Reference"=w281:refnum<vi>)
        n141 = case shown="\"Open\", Default" w280 {
          tunnel: w284 -> [w290 w303]
          tunnel: [w292 w304] -> w283
          tunnel: w281 -> [w291 w301]
          frame "Open", Default {
            n142 = property class="VI"(reference=w291, error in=w290) -> (reference out=w288:refnum<vi>, error out=w289:errorcluster, "Front Panel.Open"=w287:bool)
            n143 = case shown="False" w287 {
              tunnel: [w295 w298] -> w292
              tunnel: w289 -> [w294 w298]
              tunnel: w288 -> [w293 _]
              frame False {
                n144 = invoke class="VI" method="FP.Open"(reference=w293, error in=w294, "Activate"=TRUE, "State"=T18."Standard") -> (error out=w295:errorcluster)  [unwired: 1 in, 4 out]
              }
              frame True {
              }
            }
          }
          frame "Close" {
            n145 = property class="VI"(reference=w301, error in=w303) -> (reference out=w300:refnum<vi>, error out=w302:errorcluster, "Front Panel.Open"=w299:bool)
            n146 = case shown="True" w299 {
              tunnel: [w305 w308] -> w304
              tunnel: w302 -> [w305 w307]
              tunnel: w300 -> [_ w306]
              frame False {
              }
              frame True {
                n147 = invoke class="VI" method="FP.Close"(reference=w306, error in=w307) -> (error out=w308:errorcluster)  [unwired: 1 in, 2 out]
              }
            }
          }
        }
      }
      frame "---------- Macro ----------" {
        # "Do not put any code in this frame.\n(It is a separator no-op. You can make a copy of this frame to create a new Macro frame)"
        n148 = call <vilib>:"Add State(s) to Queue__jki_lib_state_machine.vi"("State(s) in (\"\")"=w312) -> ("States Out"=w311:string)  [unwired: 14 in]
      }
      frame "Macro: Initialize" {
        # "Initialization Macro\n(This is called once, when the VI starts)"
        n149 = call <vilib>:"Add State(s) to Queue__jki_lib_state_machine.vi"("State(s) in Front (\"\")"="Data: Initialize\nInitialize Core Data\nUI: Initialize\nUI: Get Device Name\nUI: Start SuperGUI\nUI: Front Panel State >> Open", "State(s) in (\"\")"=w317) -> ("States Out"=w316:string)  [unwired: 13 in]
      }
      frame "Macro: Exit" {
        # "Exit Macro\n(This is called once, when the VI exits)"
        n150 = Unbundle By Name(w324) -> ("Core.Close Panel on Exit?"=w323:bool)
        n151 = Select(t="UI: Front Panel State >> Close", s=w323, f="") -> (s? t:f=w320:string)
        n152 = call <vilib>:"Add State(s) to Queue__jki_lib_state_machine.vi"("State(s) in (\"\")"=w320, "State(s) at Back (\"\")"="Data: Cleanup\nExit") -> ("States Out"=w318:string)  [unwired: 13 in]
        n153 = call <vilib>:"Add State(s) to Queue__jki_lib_state_machine.vi"("State(s) in Front (\"\")"=w318, "State(s) in (\"\")"=w327) -> ("States Out"=w326:string)  [unwired: 13 in]
      }
      frame "---------- New Category ----------" {
        # "Template Separator\n(You can make a copy of, or modify, this frame)"
        n154 = call <vilib>:"Add State(s) to Queue__jki_lib_state_machine.vi"("State(s) in (\"\")"=w331) -> ("States Out"=w330:string)  [unwired: 14 in]
      }
      frame "New Category: 1" {
        # "Your code here.\n(You can make a copy of, or modify, this frame)"
        n155 = call <vilib>:"Add State(s) to Queue__jki_lib_state_machine.vi"("State(s) in (\"\")"=w335) -> ("States Out"=w334:string)  [unwired: 14 in]
      }
      frame "New Category: 2" {
        # "Your code here.\n(You can make a copy of, or modify, this frame)"
        n156 = call <vilib>:"Add State(s) to Queue__jki_lib_state_machine.vi"("State(s) in (\"\")"=w339) -> ("States Out"=w338:string)  [unwired: 14 in]
      }
    }
  }
